vi "OP600ZP_VGConf.vi"() -> ()   [LabVIEW 2020]
panel:
  out "Temps":dbl
  out "Current":dbl
  out "CBATmin":dbl
  out "DeltaU":dbl
  out "PostCurrentMax":dbl
  out "PostCurrentMin":dbl
  out "RatioUBATTOCV":dbl
  out "Relaxation":dbl
  out "Fuse_Max":dbl
  out "ZEN84_DCIR_70":dbl
  out "ZEN84_DCIR_30":dbl
  out "ZEN82_DCIR_70":dbl
  out "ZEN82_DCIR_30":dbl
  out "ZEN79_DCIR_70":dbl
  out "ZEN79_DCIR_30":dbl
  out "ZEN77_DCIR_70":dbl
  out "ZEN77_DCIR_30":dbl
  out "ZEN74_DCIR_70":dbl
  out "ZEN74_DCIR_30":dbl
  out "DeltaTCellMax0s":dbl
  out "DeltaTCellMax30s":dbl
  out "DeltaVCellMax0s":dbl
  out "DeltaVCellMax30s":dbl
  out "ZeroCurrent":dbl
  out "CBAT-":dbl
  out "CBAT+":dbl
  out "CAN_BAT_Max":dbl
  out "CAN_BAT_Min":dbl
  out "CAN_VEH_Max":dbl
  out "CAN_VEH_Min":dbl
  out "SOH":dbl
  out "SOC70Max":dbl
  out "SOC70Min":dbl
  out "SOC30Max":dbl
  out "SOC30Min":dbl
  out "DeltaV":dbl
  out "DeltaT":dbl
  out "Max":dbl
  out "ZEN84UbattMax70":dbl
  out "ZEN84UbattMin70":dbl
  out "ZEN84UbattMax30":dbl
  out "ZEN84UbattMin30":dbl
  out "ZEN82UbattMax70":dbl
  out "ZEN82UbattMin70":dbl
  out "ZEN82UbattMax30":dbl
  out "ZEN82UbattMin30":dbl
  out "ZEN79UbattMax70":dbl
  out "ZEN79UbattMin70":dbl
  out "ZEN79UbattMax30":dbl
  out "ZEN79UbattMin30":dbl
  out "ZEN77UbattMax70":dbl
  out "ZEN77UbattMin70":dbl
  out "ZEN77UbattMax30":dbl
  out "ZEN77UbattMin30":dbl
  out "ZEN74UbattMax70":dbl
  out "ZEN74UbattMin70":dbl
  out "ZEN74UbattMax30":dbl
  out "VCellMax30":dbl
  out "ZEN74UbattMin30":dbl
  out "VCellMin30":dbl
  out "VCellMax70":dbl
  out "TUsineMax":dbl
  out "VCellMin70":dbl
  out "TUsineMin":dbl
  out "TCellMax":dbl
  out "MinZEN77":dbl
  out "TCellMin":dbl
  out "IsoMin":dbl
  out "PDU-":dbl
  out "Rmin":dbl
  out "PDU+":dbl
  out "Rmax":dbl
  in  "3562":string
  in  "MX5060":string
  in  "ST5520":string
  # "[EQUIPEMENT]\nST5520 = HIOKI,ST5520,221163897,V2.04\t\nMX5060 = B\n3562 = HIOKI,BT3562A,0,V2.01\n\n[Conti]\nRmax = 1\n\n[Iso]\nIsoMin = 16.7\nMinZEN77 = 4.5\nPDU+ = 25\nPDU- = 18\n\n[DataDyn]\nTCellMin = 16\nTCellMax = 32\nTusineMin = 16\nTusineMax = 32\nVCellMin30 = 3400\nVCellMax30 = 3700\nVCellMin70 = 3700\nVCellMax70 = 4000\nZEN74UbattMax30 = 620\nZEN74UbattMin30 = 589\nZEN74UbattMax70 = 663\nZEN74UbattMin70 = 651\nZEN77UbattMax30 = 642\nZEN77UbattMin30 = 610\nZEN77UbattMax70 = 687\nZEN77UbattMin70 = 675\nZEN79UbattMax30 = 665\nZEN79UbattMin30 = 631\nZEN79UbattMax70 = 711\nZEN79UbattMin70 = 698\nZEN82UbattMax30 = 688\nZEN82UbattMin30 = 652\nZEN82UbattMax70 = 734\nZEN82UbattMin70 = 721\nZEN84UbattMax30 = 673\nZEN84UbattMin30 = 710\nZEN84UbattMax70 = 758\nZEN84UbattMin70 = 745\nDeltaT = 3\nDeltaV = 30\nSOC30Min = 20\nSOC30Max = 40\nSOC70Min = 60\nSOC70Max = 80\nSOH = 97\n\n[Sealing]\nMax = 200\n\n[OCVACIR]\nZEN74ACIR = 92.5\nZEN77ACIR = 95.3\nZEN79ACIR = 98.0\nZEN82ACIR = 100.8\nZEN84ACIR = 103.5\n\n[CMU]\nZEN74TEMP = 56\nZEN74TENS = 168\nZEN77TEMP = 58\nZEN77TENS = 174\nZEN79TEMP = 60\nZEN79TENS = 180\nZEN82TEMP = 62\nZEN82TENS = 186\nZEN84TEMP = 64\nZEN84TENS = 192"
  # "EQUIPEMENTS"
  # "Conti"
  # "Iso"
  # "Sealing"
  # "DataDyn"
  # "DCIR"
  # "PRECHARGE"
  # "CAPACITE"
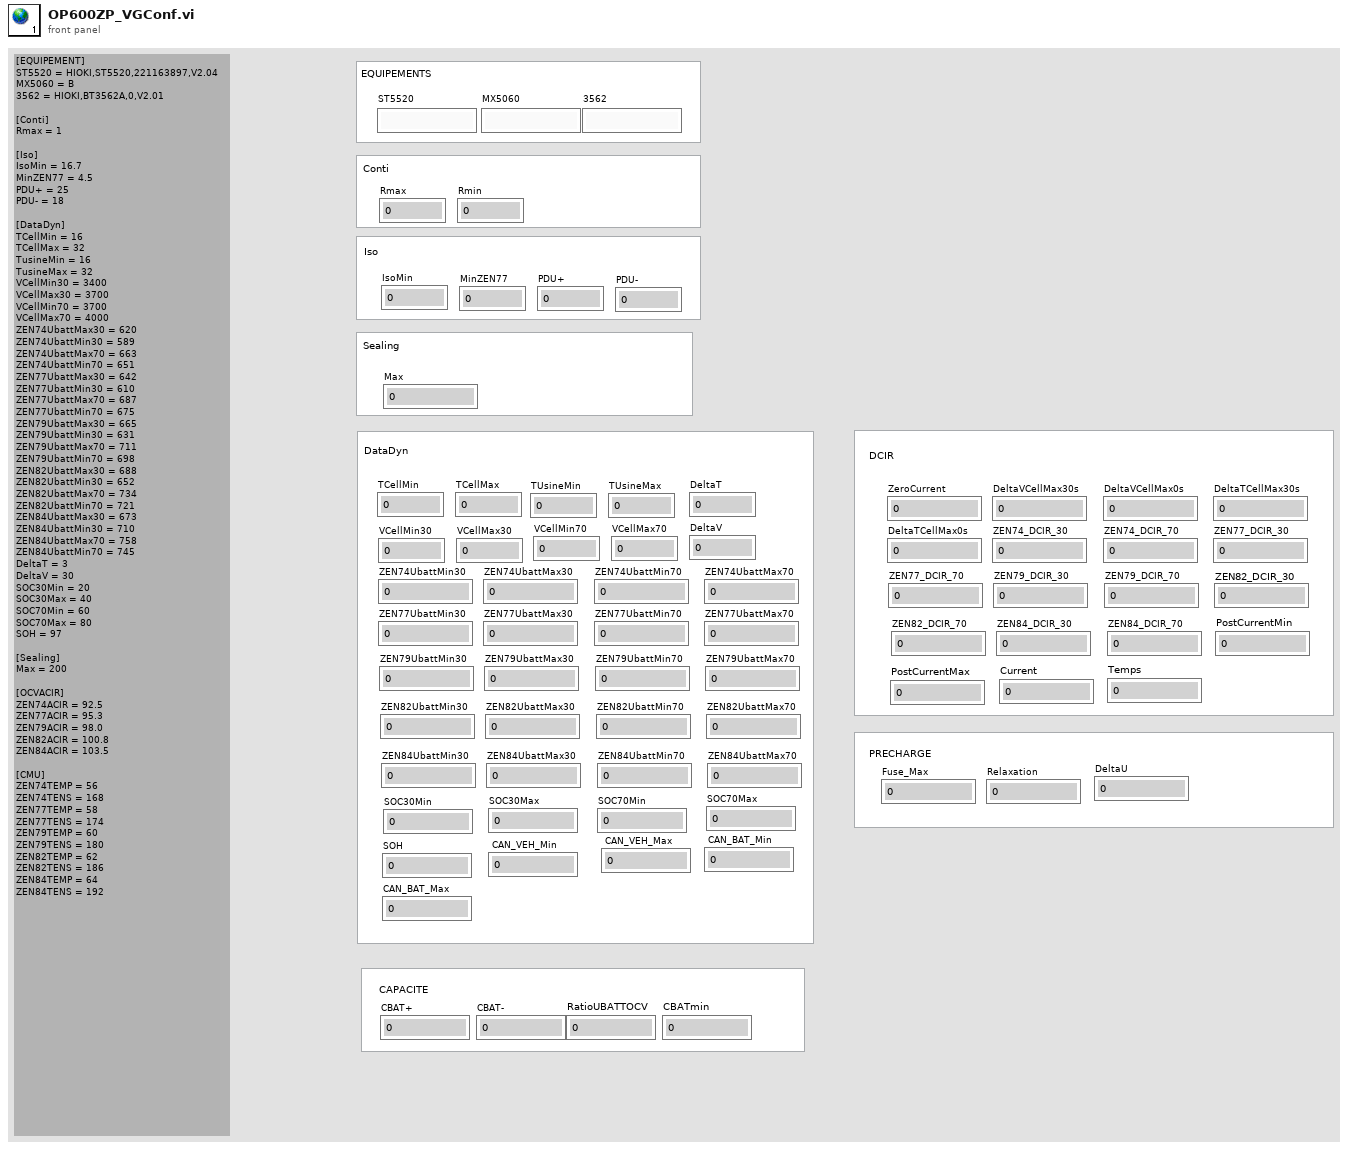
[diagram p1: front panel]
diagram:
